vi "Launch Wizard.vi"(8 "error in (no error)":errorcluster, 10 "Controller in":refnum<class "Controller.lvclass">, 11 "New Project Wizard in":refnum<class "New Project Wizard.lvclass">) -> (0 "error out":errorcluster, 3 "Caller-To-Actor Enqueuer":refnum<class "Message Enqueuer.lvclass">)   [LabVIEW 2013, in "SET Project Editor.lvlib" / "New Project Wizard.lvclass"]
uses:
  New Project Wizard.lvclass
  <vilib>/ActorFramework/Message Enqueuer/Message Enqueuer.lvclass
  controller/Controller.lvclass
  controller/Controller.lvclass/Controller.ctl
  New Project Wizard.lvclass/New Project Wizard.ctl
  UI Wizard/UI Wizard.lvclass
  controller/Read Default Path.vi
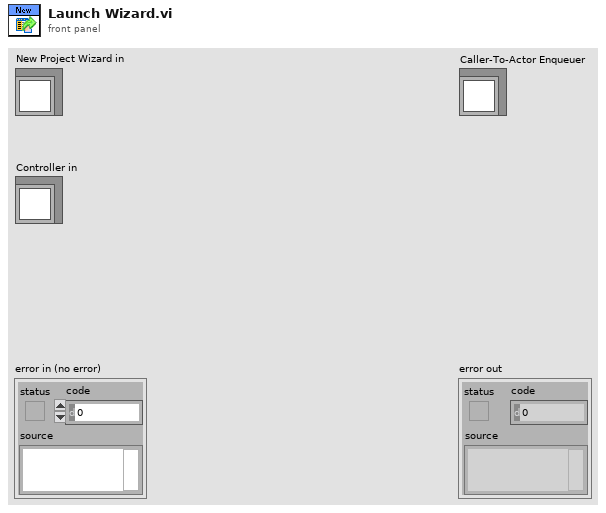
[diagram p1: front panel]
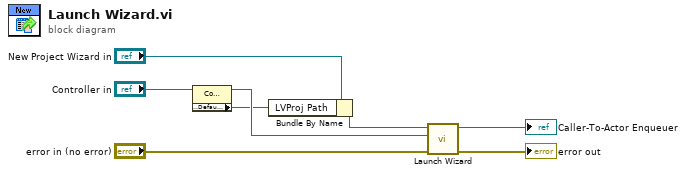
[diagram p0: block diagram]
diagram:
  n1 = property class="Controller.lvclass"(reference="Controller in") -> (reference out=w4:refnum<class "Controller.lvclass">, "Properties:Default Path"=w1:path)  [unwired: 1 in, 1 out]
  n2 = Bundle By Name(cluster="New Project Wizard in", "LVProj Path"=w1) -> (w2:refnum<class "New Project Wizard.lvclass">)
  n3 = call-parent "Launch Wizard.vi"("error in (no error)"="error in (no error)", "Controller in"=w4, "UI Wizard in"=w2) -> ("error out"=→"error out":errorcluster, "Caller-To-Actor Enqueuer"=→"Caller-To-Actor Enqueuer":refnum<class "Message Enqueuer.lvclass">)  [unwired: 7 in]
